vi "clearTCPBuffer.vi"(9 "data in":string, 11 "connection ID":refnum<k5>) -> (1 "data out":string, 3 "connection ID out":refnum<k5>)   [LabVIEW 2009]
panel:
  out "data out 2":string
  out "Numeric":i32
  out "error IO":errorcluster
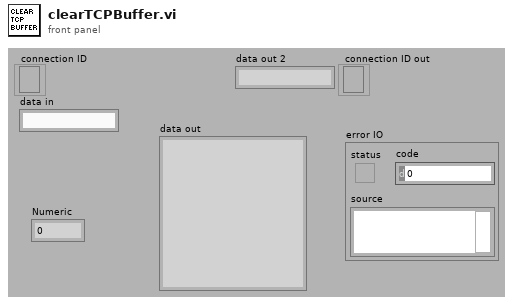
[diagram p1: front panel]
types:
  T1 = enum16{"Standard", "Buffered", "CRLF", "Immediate"}
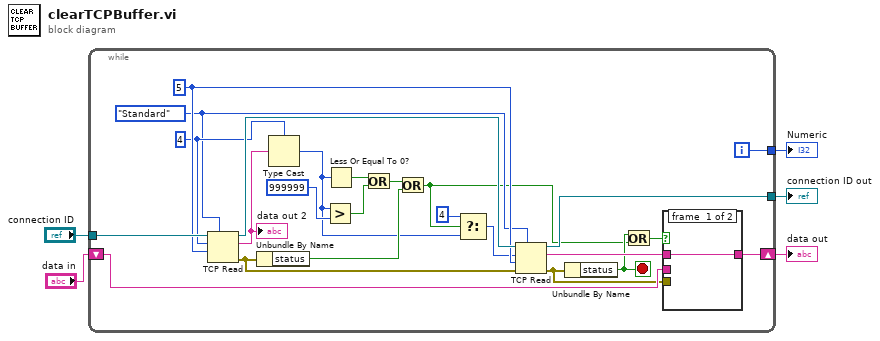
[diagram p0: block diagram]
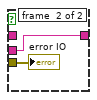
[diagram p2: hidden frame]
diagram:
  n1 = while {
    tunnel: "connection ID" -> [w28]
    tunnel: [w27] -> w4
    shift-right: [w25] -> w2
    shift-left: "data in" -> [w24]
    tunnel: [w23] -> w1
    i -> [w23]
    stop <- w9 stop-if-true
    w10 = T1."Standard" ("mode (standard)")
    w26 = 5 ("timeout ms (25000)")
    w21 = 4
    n2 = TCP Read(connection ID=w28, bytes to read=w21, 7:w10, 9:w26) -> (connection ID out=w29:refnum<k5>, data out=w22:string, error out=w17:errorcluster)  [unwired: 1 in]
    "data out 2" <- w22
    n3 = Unbundle By Name(w17) -> ("status"=w15:bool)
    n4 = Type Cast(type=w21, x=w22) -> (*(type *) &x=w13:i32)
    n5 = Greater?(x=w13, y=999999) -> (0:w18:bool)
    n6 = Less Or Equal To 0?(x=w13) -> (x <= 0?=w19:bool)
    n7 = Or(x=w19, y=w18) -> (x .or. y?=w16:bool)
    n8 = Or(x=w16, y=w15) -> (x .or. y?=w8:bool)
    n9 = Select(t=4, s=w8, f=w13) -> (s? t:f=w11:i32)
    n10 = TCP Read(connection ID=w29, bytes to read=w11, error in (no error)=w17, 7:w10, 9:w26) -> (connection ID out=w27:refnum<k5>, data out=w14:string, error out=w6:errorcluster)
    n11 = Unbundle By Name(w6) -> ("status"=w9:bool)
    n12 = Or(x=w9, y=w8) -> (x .or. y?=w7:bool)
    n13 = case shown="True" w7 {
      tunnel: [w30 w32] -> w25
      tunnel: w14 -> [w30 _]
      tunnel: w24 -> [_ w32]
      tunnel: w6 -> [_ w31]
      frame #0 {
      }
      frame #1 {
        "error IO" <- w31
      }
    }
  }
  "connection ID out" <- w4
  "data out" <- w2
  "Numeric" <- w1
